vi "Read (Math).vi"(0 "VISA resource name":refnum<visa-resource-name>, 11 "error in (no error)":errorcluster) -> (3 "Measurement Count":dbl, 4 "VISA resource name out":refnum<visa-resource-name>, 6 "Minimum Value":dbl, 8 "Maximum Value":dbl, 10 "Average":dbl, 13 "Standard Deviation":dbl, 14 "Peak to Peak Measurement":dbl, 15 "error out":errorcluster)   [LabVIEW 2022 SP3, in "Agilent 34420.lvlib"]
doc: "Reads and returns the math statistics measurement results."
uses:
  Agilent 34420.lvlib
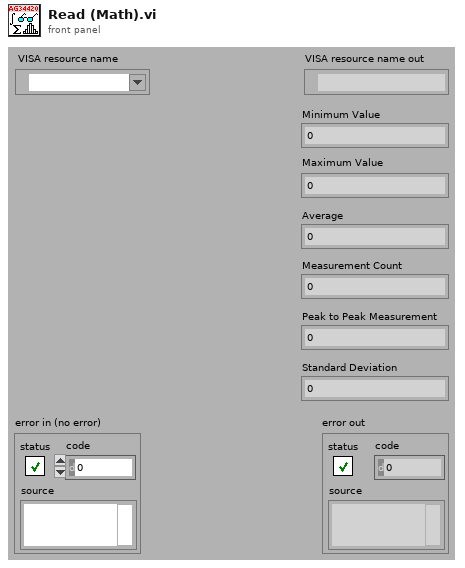
[diagram p1: front panel]
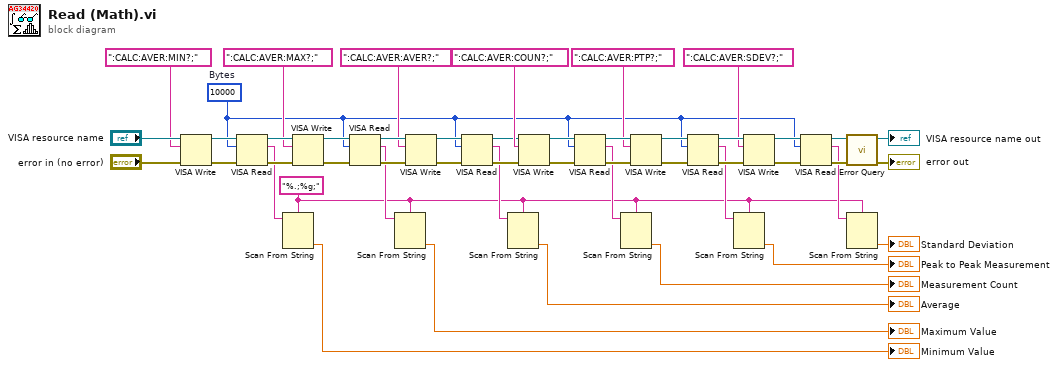
[diagram p0: block diagram]
diagram:
  w7 = "%.;%g;" ("format string")
  w14 = u32 10000  # Bytes
  n1 = VISA Write(VISA resource name="VISA resource name", write buffer=":CALC:AVER:MIN?;", error in (no error)="error in (no error)") -> (VISA resource name out=w47:refnum<visa-resource-name>, error out=w48:errorcluster)  [unwired: 1 out]
  n2 = VISA Read(VISA resource name=w47, byte count=w14, error in (no error)=w48) -> (VISA resource name out=w36:refnum<visa-resource-name>, read buffer=w13:string, error out=w28:errorcluster)  [unwired: 1 out]
  n3 = Scan From String(format string=w7, input string=w13) -> (output 1=→"Minimum Value":dbl)  [unwired: 3 in, 3 out]
  n4 = VISA Write(VISA resource name=w36, write buffer=":CALC:AVER:MAX?;", error in (no error)=w28) -> (VISA resource name out=w35:refnum<visa-resource-name>, error out=w27:errorcluster)  [unwired: 1 out]
  n5 = VISA Read(VISA resource name=w35, byte count=w14, error in (no error)=w27) -> (VISA resource name out=w34:refnum<visa-resource-name>, read buffer=w12:string, error out=w26:errorcluster)  [unwired: 1 out]
  n6 = Scan From String(format string=w7, input string=w12) -> (output 1=→"Maximum Value":dbl)  [unwired: 3 in, 3 out]
  n7 = VISA Write(VISA resource name=w34, write buffer=":CALC:AVER:AVER?;", error in (no error)=w26) -> (VISA resource name out=w33:refnum<visa-resource-name>, error out=w25:errorcluster)  [unwired: 1 out]
  n8 = VISA Read(VISA resource name=w33, byte count=w14, error in (no error)=w25) -> (VISA resource name out=w17:refnum<visa-resource-name>, read buffer=w11:string, error out=w41:errorcluster)  [unwired: 1 out]
  n9 = Scan From String(format string=w7, input string=w11) -> (output 1=→"Average":dbl)  [unwired: 3 in, 3 out]
  n10 = VISA Write(VISA resource name=w17, write buffer=":CALC:AVER:COUN?;", error in (no error)=w41) -> (VISA resource name out=w32:refnum<visa-resource-name>, error out=w24:errorcluster)  [unwired: 1 out]
  n11 = VISA Read(VISA resource name=w32, byte count=w14, error in (no error)=w24) -> (VISA resource name out=w39:refnum<visa-resource-name>, read buffer=w10:string, error out=w40:errorcluster)  [unwired: 1 out]
  n12 = Scan From String(format string=w7, input string=w10) -> (output 1=→"Measurement Count":dbl)  [unwired: 3 in, 3 out]
  n13 = VISA Write(VISA resource name=w39, write buffer=":CALC:AVER:PTP?;", error in (no error)=w40) -> (VISA resource name out=w31:refnum<visa-resource-name>, error out=w23:errorcluster)  [unwired: 1 out]
  n14 = VISA Read(VISA resource name=w31, byte count=w14, error in (no error)=w23) -> (VISA resource name out=w37:refnum<visa-resource-name>, read buffer=w9:string, error out=w38:errorcluster)  [unwired: 1 out]
  n15 = Scan From String(format string=w7, input string=w9) -> (output 1=→"Peak to Peak Measurement":dbl)  [unwired: 3 in, 3 out]
  n16 = VISA Write(VISA resource name=w37, write buffer=":CALC:AVER:SDEV?;", error in (no error)=w38) -> (VISA resource name out=w30:refnum<visa-resource-name>, error out=w22:errorcluster)  [unwired: 1 out]
  n17 = VISA Read(VISA resource name=w30, byte count=w14, error in (no error)=w22) -> (VISA resource name out=w29:refnum<visa-resource-name>, read buffer=w8:string, error out=w21:errorcluster)  [unwired: 1 out]
  n18 = call "Error Query.vi"("error in (no error)"=w21, "VISA resource name"=w29) -> ("error out"=→"error out":errorcluster, "VISA resource name out"=→"VISA resource name out":refnum<visa-resource-name>)  [unwired: 6 in, 2 out]
  n19 = Scan From String(format string=w7, input string=w8) -> (output 1=→"Standard Deviation":dbl)  [unwired: 3 in, 3 out]
